vi "chartsheet set chart.vi"(8 "error in (no error)":errorcluster, 10 "chart":u32, 11 "chartsheet":u32) -> (0 "error out":errorcluster, 3 "function return":u32(ring))   [LabVIEW 2015, in "xlsxwriter.lvlib"]
doc: "lxw_error chartsheet_set_chart(lxw_chartsheet chartsheet, lxw_chart chart);"
uses:
  xlsxwriter.lvlib
  xlsxwriter.dll
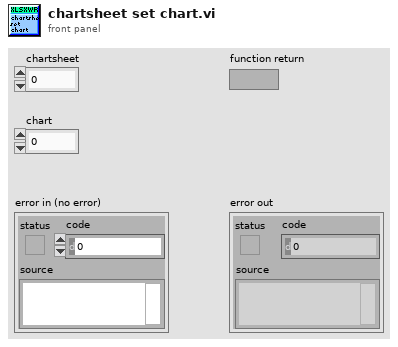
[diagram p1: front panel]
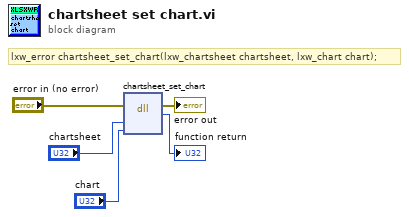
[diagram p0: block diagram]
diagram:
  # "lxw_error chartsheet_set_chart(lxw_chartsheet chartsheet, lxw_chart chart);"
  n1 = dll-call lib="C:/Users/WDAGUtilityAccount/Desktop/lv_vis_added_cell/xlsxwriter.*" fn="chartsheet_set_chart"(error in="error in (no error)", "chartsheet"="chartsheet", "chart"="chart") -> (error out=→"error out":errorcluster, →"function return":u32)  [unwired: 4 in, 1 out]
